vi "Translate Lamp Data.vi"(11 "Lamp":T2) -> (3 "output lamp message":T1)   [LabVIEW 2016]
uses:
  Lamp Data.ctl
  Messages/Lamp Message Struct.ctl
  Libs/Messages.lvlib
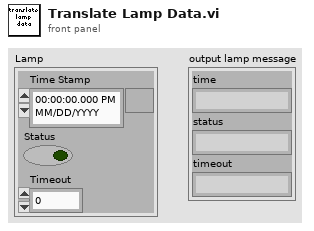
[diagram p1: front panel]
types:
  T1 = typedef "Messages.lvlib/Lamp Message Struct.ctl" = cluster{"time":string, "status":string, "timeout":string}
  T2 = typedef "Lamp Data.ctl" = cluster{"Time Stamp":timestamp, "Status":bool, "Timeout":dbl}
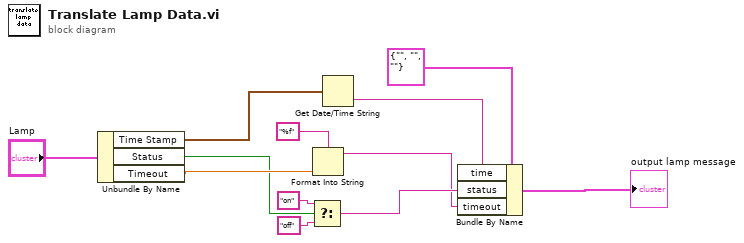
[diagram p0: block diagram]
diagram:
  n1 = Unbundle By Name("Lamp") -> ("Time Stamp"=w7:timestamp, "Status"=w5:bool, "Timeout"=w6:dbl)
  n2 = Select(t="on", s=w5, f="off") -> (s? t:f=w10:string)
  n3 = Format Into String(format string="%f", w6) -> (resulting string=w9:string)  [unwired: 2 in, 1 out]
  n4 = Get Date/Time String(seconds (now)=w7) -> (time string=w11:string)  [unwired: 2 in, 1 out]
  n5 = Bundle By Name(cluster=T1 {"time"="", "status"="", "timeout"=""}, "time"=w11, "status"=w10, "timeout"=w9) -> (→"output lamp message":T1)
